vi "Decode PNG pHYs Chunk.vi"(10 "error in (no error)":errorcluster, 11 "data":u8[](array[numeric])) -> (2 "error out":errorcluster, 3 "Pixel Dimension":T1)   [LabVIEW 2021, in "Files.lvlib"]
uses:
  Files.lvlib
  PNG Pixel Dimension.ctl
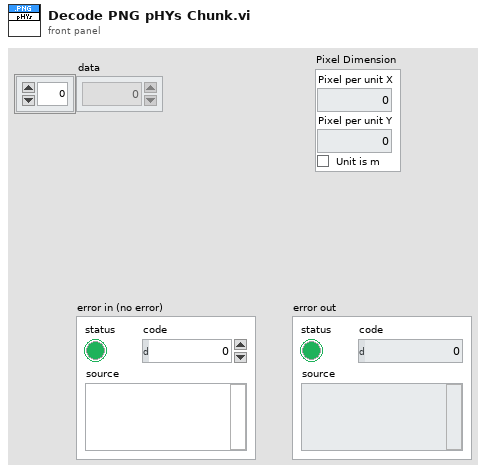
[diagram p1: front panel]
types:
  T1 = typedef "Files.lvlib/PNG Pixel Dimension.ctl" = cluster{"Pixel per unit X":u32, "Pixel per unit Y":u32, "Unit is m":bool}
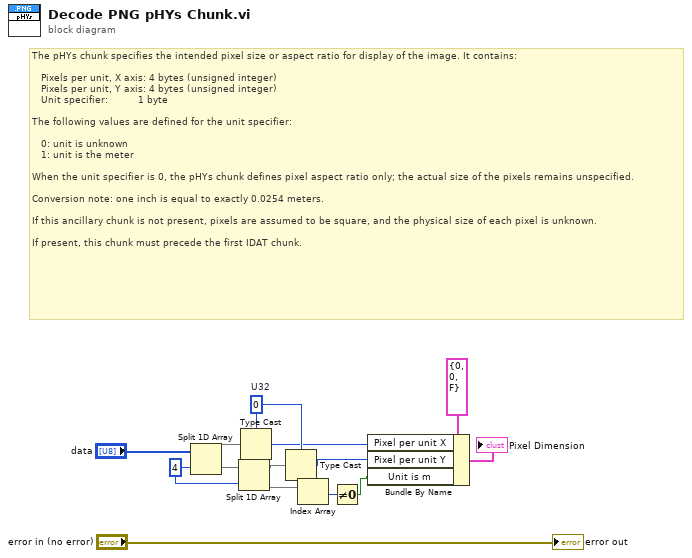
[diagram p0: block diagram]
diagram:
  w7 = u32 0  # U32
  w11 = 4 ("index")
  # "The pHYs chunk specifies the intended pixel size or aspect ratio for display of the image. It contains:\n\n   Pixels per unit, X axis: 4 bytes (unsigned integer)\n   Pixels per unit, Y axis: 4 bytes (unsigned integer)\n   Unit specifier:          1 byte\n\nThe following values are defined for the unit specifier:\n\n   0: unit is unknown\n   1: unit is the meter\n\nWhen the unit specifier is 0, the pHYs chunk defines pixel aspect ratio only; the actual size of the pixels remains unspecified.\n\nConversion note: one inch is equal to exactly 0.0254 meters.\n\nIf this ancillary chunk is not present, pixels are assumed to be square, and the physical size of each pixel is unknown.\n\nIf present, this chunk must precede the first IDAT chunk."
  n1 = Split 1D Array(array="data", index=w11) -> (first subarray=w9:u8[], second subarray=w12:u8[])
  n2 = Split 1D Array(array=w12, index=w11) -> (first subarray=w8:u8[], second subarray=w10:u8[])
  n3 = Type Cast(type=w7, x=w9) -> (*(type *) &x=w4:u32)
  n4 = Type Cast(type=w7, x=w8) -> (*(type *) &x=w3:u32)
  n5 = Index Array(array=w10) -> (element=w2:u8)  [unwired: 1 in]
  n6 = Not Equal To 0?(x=w2) -> (x != 0?=w1:bool)
  n7 = Bundle By Name(cluster=T1 {"Pixel per unit X"=0, "Pixel per unit Y"=0, "Unit is m"=FALSE} ("Pixel Dimension"), "Pixel per unit X"=w4, "Pixel per unit Y"=w3, "Unit is m"=w1) -> (→"Pixel Dimension":T1)
  "error out" <- "error in (no error)"
